vi "Rinse.vi"(8 "High pressure purge time (s)":dbl=30.0 format="%#.4f", 9 "High pressure purge?":bool=TRUE, 10 "Control parameters":T1={"Pump 2 fill rate (ml/min)"=0.5, "Pump 2 rinse times"=2, "Pump 2 fill volume (ml)"=0.015, "Pump 1 rinse rate (ml/min)"=0.2, "Pump 1 rinse volume (mL)"=1.0, "Pump 1 fill volume (mL)"=1.0, "Pump 1 fill rate (ml/min)"=3.0, "Delayed time for waiting(s)"=5.0, "Pump 3 fill rate (ml/min)"=0.5, "Pump 3 fill volume (ml)"=0.015, "Pump 3 muliplier"=1.2, "Pump 3 rinse times"=1, "Gas purge muliplier"=2.0, "Gas purge?"=TRUE, "Pump 1 clear rate (ml/min)"=0.1, "Clear?"=TRUE, "Rinse injection order"=enum."Pump 2 first"} {"Pump 1 clear rate (ml/min)" format="%#.4f"; "Gas purge muliplier" min=0.0 max=50.0 format="%#.3g"; "Pump 3 muliplier" min=0.0 max=50.0 format="%#.3g"; "Pump 3 fill volume (ml)" min=0.0 max=50.0 format="%#.3g"; "Pump 3 fill rate (ml/min)" min=0.0 max=500.0 format="%#.3g"; "Pump 1 fill rate (ml/min)" format="%#.4f"; "Pump 1 fill volume (mL)" format="%#.4f"; "Pump 1 rinse volume (mL)" format="%#.4f"; "Pump 1 rinse rate (ml/min)" format="%#.4f"; "Pump 2 fill volume (ml)" min=0.0 max=50.0 format="%#.3g"; "Pump 2 fill rate (ml/min)" min=0.0 max=500.0 format="%#.3g"}, 11 "Configured COM ports":T2={"Pump 1 COM"="COM12", "Pump 2 COM"="COM9", "Pump 3 COM"="COM13", "Pump 4 COM"="COM4", "Pump 5 COM"="COM15"}) -> ()   [LabVIEW 2017]
uses:
  <instrlib>/Harvard Apparatus PHD Ultra Series/Harvard Apparatus PHD Ultra Series.lvlib
  <instrlib>/Harvard Syringe Pump PHD2000/Harvard Syringe Pump PHD2000.lvlib
panel:
  out "Rinse injection order":enum16{"Pump 2 first", "Pump 3 first"}(ring)
  out "Clear?":bool
  out "Pump 1 clear rate (ml/min)":dbl=0.6 format="%#.4f"
  out "Gas purge?":bool
  out "Gas purge muliplier":dbl=1.2 min=0.0 max=50.0 format="%#.3g"
  out "Pump 3 rinse times":i32=2
  out "Pump 3 muliplier":dbl=1.2 min=0.0 max=50.0 format="%#.3g"
  out "Rinse injection selector":enum16{"Pump 2", "Pump 3"}(ring)
  out "Pump 3 fill volume (ml)":dbl=0.1 min=0.0 max=50.0 format="%#.3g"
  out "Pump 3 fill rate (ml/min)":dbl=0.5 min=0.0 max=500.0 format="%#.3g"
  out "Pump 5 COM":refnum<visa-resource-name>="COM12"
  out "Pump 1 rinse volume (mL)":dbl=0.4 format="%#.4f"
  out "Pump 1 rinse rate (ml/min)":dbl=0.6 format="%#.4f"
  out "Delayed time for waiting(s)":dbl
  out "Pump 1 fill volume (mL)":dbl=0.4 format="%#.4f"
  out "Pump 1 fill rate (ml/min)":dbl=1.5 format="%#.4f"
  out "Counter":i32
  out "Action selector":enum16{"Fill", "Rinse", "Clear"}(ring)
  out "Pump 2 rinse times":i32=2
  out "Pump 2 fill volume (ml)":dbl=0.1 min=0.0 max=50.0 format="%#.3g"
  out "Pump 2 fill rate (ml/min)":dbl=0.5 min=0.0 max=500.0 format="%#.3g"
  out "Pump 4 COM":refnum<visa-resource-name>="COM12"
  out "Pump 3 COM":refnum<visa-resource-name>="COM12"
  out "Pump 2 COM":refnum<visa-resource-name>="COM12"
  out "Pump 1 COM":refnum<visa-resource-name>="COM12"
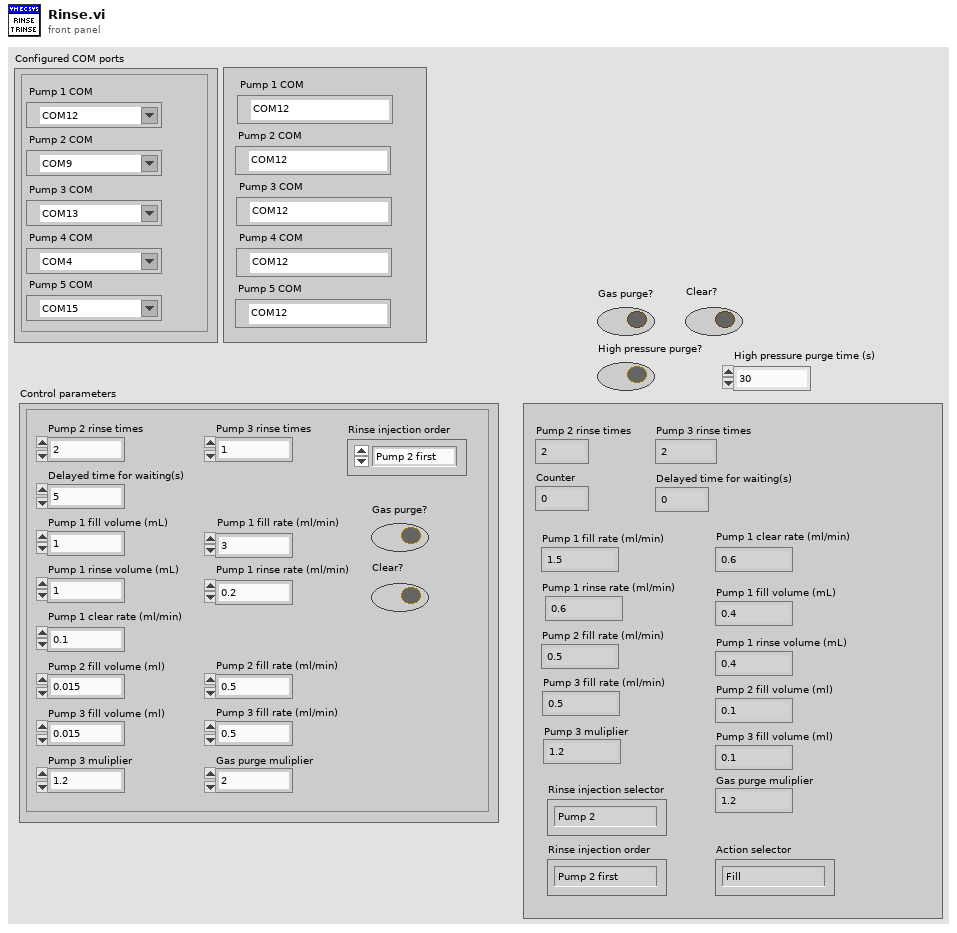
[diagram p1: front panel]
types:
  T1 = cluster{"Pump 2 fill rate (ml/min)":dbl, "Pump 2 rinse times":i32, "Pump 2 fill volume (ml)":dbl, "Pump 1 rinse rate (ml/min)":dbl, "Pump 1 rinse volume (mL)":dbl, "Pump 1 fill volume (mL)":dbl, "Pump 1 fill rate (ml/min)":dbl, "Delayed time for waiting(s)":dbl, "Pump 3 fill rate (ml/min)":dbl, "Pump 3 fill volume (ml)":dbl, "Pump 3 muliplier":dbl, "Pump 3 rinse times":i32, "Gas purge muliplier":dbl, "Gas purge?":bool, "Pump 1 clear rate (ml/min)":dbl, "Clear?":bool, "Rinse injection order":enum16{"Pump 2 first", "Pump 3 first"}}
  T2 = cluster{"Pump 1 COM":refnum<visa-resource-name>, "Pump 2 COM":refnum<visa-resource-name>, "Pump 3 COM":refnum<visa-resource-name>, "Pump 4 COM":refnum<visa-resource-name>, "Pump 5 COM":refnum<visa-resource-name>}
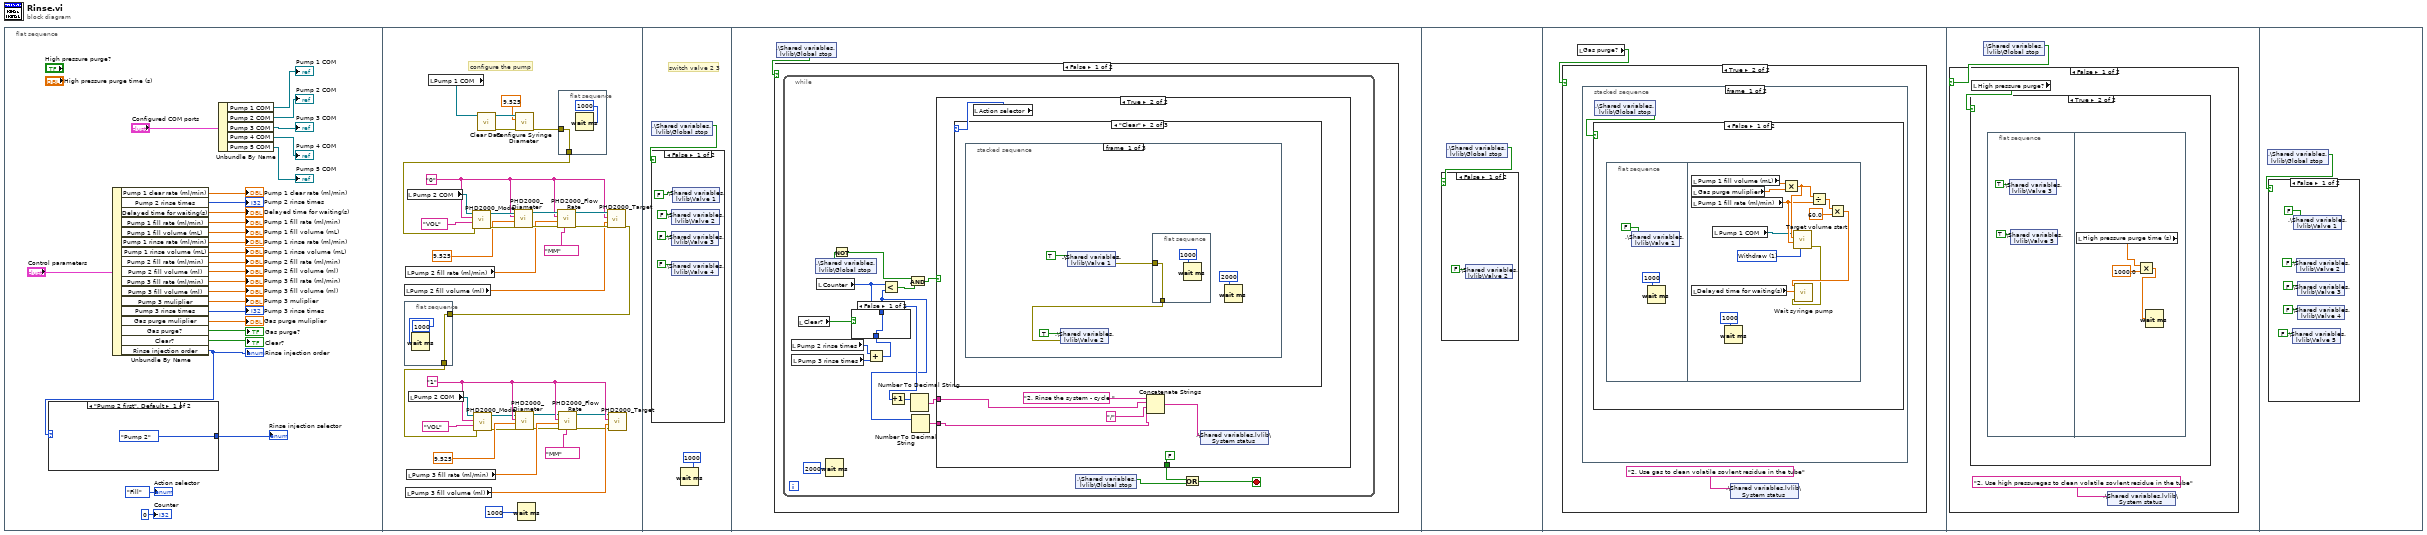
[diagram p0: block diagram]
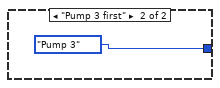
[diagram p2: hidden frame]
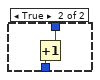
[diagram p4: hidden frame]
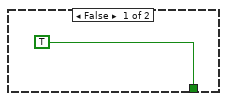
[diagram p5: hidden frame]
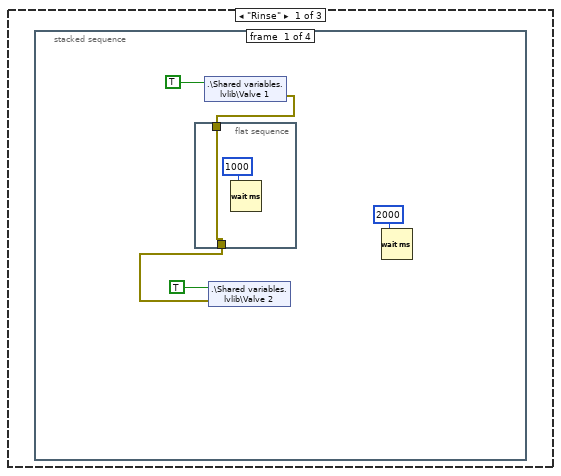
[diagram p6: hidden frame]
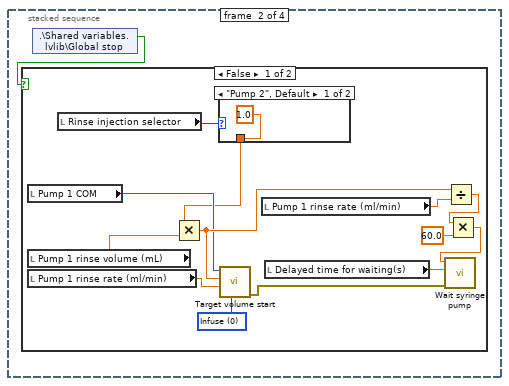
[diagram p7: hidden frame]
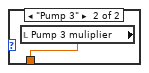
[diagram p8: hidden frame]
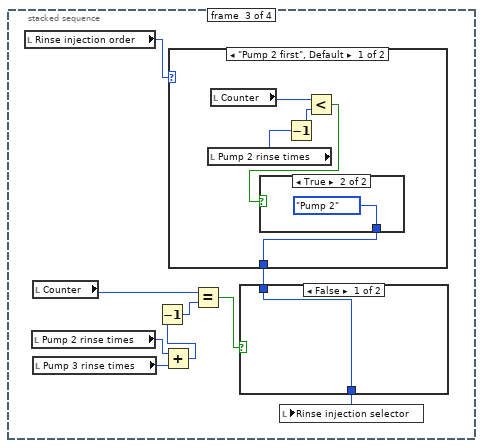
[diagram p10: hidden frame]
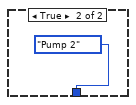
[diagram p11: hidden frame]
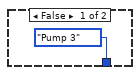
[diagram p12: hidden frame]
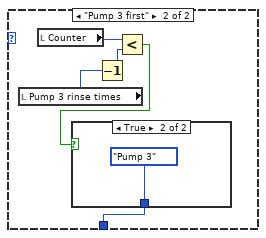
[diagram p13: hidden frame]
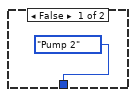
[diagram p14: hidden frame]
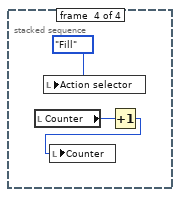
[diagram p15: hidden frame]
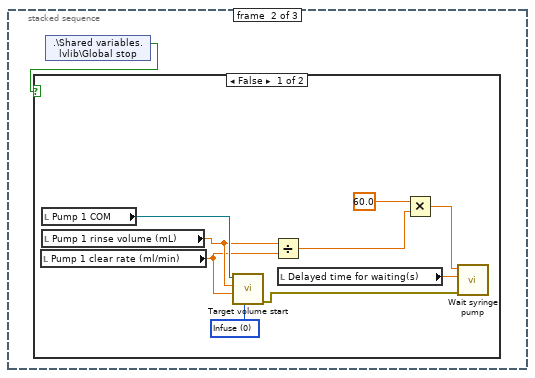
[diagram p16: hidden frame]
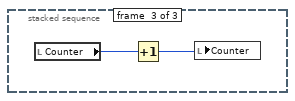
[diagram p18: hidden frame]
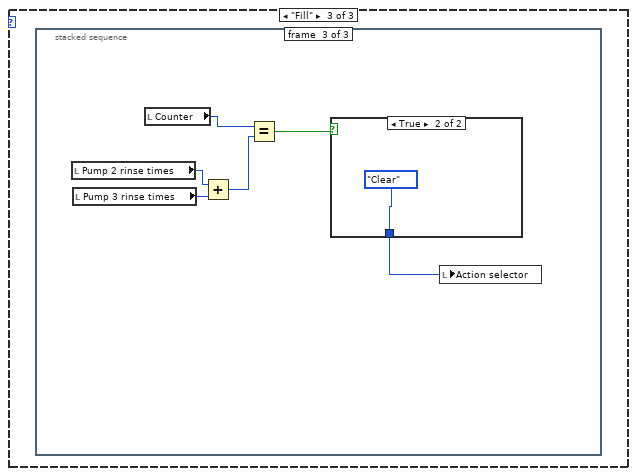
[diagram p19: hidden frame]
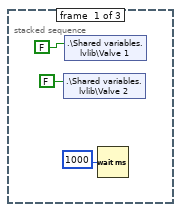
[diagram p20: hidden frame]
diagram:
  n1 = flat-sequence {
    frame #0 {
      n2 = Unbundle By Name("Control parameters") -> ("Pump 1 clear rate (ml/min)"=→"Pump 1 clear rate (ml/min)":dbl, "Pump 2 rinse times"=→"Pump 2 rinse times":i32, "Delayed time for waiting(s)"=→"Delayed time for waiting(s)":dbl, "Pump 1 fill rate (ml/min)"=→"Pump 1 fill rate (ml/min)":dbl, "Pump 1 fill volume (mL)"=→"Pump 1 fill volume (mL)":dbl, "Pump 1 rinse rate (ml/min)"=→"Pump 1 rinse rate (ml/min)":dbl, "Pump 1 rinse volume (mL)"=→"Pump 1 rinse volume (mL)":dbl, "Pump 2 fill rate (ml/min)"=→"Pump 2 fill rate (ml/min)":dbl, "Pump 2 fill volume (ml)"=→"Pump 2 fill volume (ml)":dbl, "Pump 3 fill rate (ml/min)"=→"Pump 3 fill rate (ml/min)":dbl, "Pump 3 fill volume (ml)"=→"Pump 3 fill volume (ml)":dbl, "Pump 3 muliplier"=→"Pump 3 muliplier":dbl, "Pump 3 rinse times"=→"Pump 3 rinse times":i32, "Gas purge muliplier"=→"Gas purge muliplier":dbl, "Gas purge?"=→"Gas purge?":bool, "Clear?"=→"Clear?":bool, "Rinse injection order"=w1:enum16{"Pump 2 first", "Pump 3 first"})
      "Rinse injection order" <- w1
      n3 = case shown="\"Pump 2 first\", Default" w1 {
        tunnel: [enum16{"Pump 2", "Pump 3"}."Pump 2" ("Rinse injection selector") enum16{"Pump 2", "Pump 3"}."Pump 3" ("Rinse injection selector")] -> w2
        frame "Pump 2 first", Default {
        }
        frame "Pump 3 first" {
        }
      }
      "Rinse injection selector" <- w2
      n4 = Unbundle By Name("Configured COM ports") -> ("Pump 1 COM"=→"Pump 1 COM":refnum<visa-resource-name>, "Pump 2 COM"=→"Pump 2 COM":refnum<visa-resource-name>, "Pump 3 COM"=→"Pump 3 COM":refnum<visa-resource-name>, "Pump 4 COM"=→"Pump 4 COM":refnum<visa-resource-name>, "Pump 5 COM"=→"Pump 5 COM":refnum<visa-resource-name>)
      "Action selector" <- enum16{"Fill", "Rinse", "Clear"}."Fill" ("Action selector")
      "Counter" <- 0 ("Counter")
    }
    frame #1 {
      w41 = "1" ("Pump #")
      w50 = "0" ("Pump #")
      # "configure the pump"
      n5 = local read "Pump 2 fill volume (ml)"() -> (w48:dbl)
      n6 = flat-sequence {
        tunnel: w44 -> [w65]
        tunnel: [w65] -> w30
        frame #0 {
          n7 = Wait (ms)(milliseconds to wait=u32 1000) -> ()  [unwired: 1 out]
        }
      }
      n8 = local read "Pump 2 fill rate (ml/min)"() -> (w49:dbl)
      n9 = local read "Pump 3 fill volume (ml)"() -> (w43:dbl)
      n10 = local read "Pump 3 fill rate (ml/min)"() -> (w42:dbl)
      n11 = local read "Pump 2 COM"() -> (w55:refnum<visa-resource-name>)
      n12 = local read "Pump 2 COM"() -> (w36:refnum<visa-resource-name>)
      n13 = local read "Pump 1 COM"() -> (w57:refnum<visa-resource-name>)
      n14 = call <instrlib>:"PHD2000_Mode.vi"("error in (no error)"=w46, "Mode"="VOL", "Pump #"=w50, "VISA resource name 2"=w55) -> ("error out"=w53:errorcluster, "VISA resource name out"=w54:refnum<visa-resource-name>)  [unwired: 5 in, 1 out]
      n15 = call <instrlib>:"PHD2000_Mode.vi"("error in (no error)"=w30, "Mode"="VOL", "Pump #"=w41, "VISA resource name 2"=w36) -> ("error out"=w38:errorcluster, "VISA resource name out"=w37:refnum<visa-resource-name>)  [unwired: 5 in, 1 out]
      n16 = call <instrlib>:"Clear Data.vi"("VISA resource name"=w57) -> ("error out"=w59:errorcluster, "VISA resource name out"=w58:refnum<visa-resource-name>)  [unwired: 9 in]
      n17 = call <instrlib>:"PHD2000_Diameter.vi"("VISA resource name 2"=w54, "Pump #"=w50, "diameter (mm)"=9.525 ("Syringe Diameter (20 mm)"), "error in (no error)"=w53) -> ("VISA resource name out"=w61:refnum<visa-resource-name>, "error out"=w63:errorcluster)  [unwired: 5 in]
      n18 = call <instrlib>:"Configure Syringe Diameter.vi"("error in (no error)"=w59, "Syringe Diameter (20 mm)"=9.525, "VISA resource name"=w58) -> ("error out"=w45:errorcluster)  [unwired: 7 in, 1 out]
      n19 = call <instrlib>:"PHD2000_Diameter.vi"("VISA resource name 2"=w37, "Pump #"=w41, "diameter (mm)"=9.525 ("Syringe Diameter (20 mm)"), "error in (no error)"=w38) -> ("VISA resource name out"=w34:refnum<visa-resource-name>, "error out"=w32:errorcluster)  [unwired: 5 in]
      n20 = Wait (ms)(milliseconds to wait=u32 1000) -> ()  [unwired: 1 out]
      n21 = call <instrlib>:"PHD2000_Flow Rate.vi"("VISA resource name 2"=w61, "Pump #"=w50, "flowrate"=w49, "error in (no error)"=w63, "Unit"="MM") -> ("VISA resource name out"=w62:refnum<visa-resource-name>, "error out"=w64:errorcluster)  [unwired: 4 in]
      n22 = flat-sequence {
        tunnel: [w67] -> w46
        tunnel: w45 -> [w67]
        frame #0 {
          n23 = Wait (ms)(milliseconds to wait=u32 1000) -> ()  [unwired: 1 out]
        }
      }
      n24 = call <instrlib>:"PHD2000_Flow Rate.vi"("VISA resource name 2"=w34, "Pump #"=w41, "flowrate"=w42, "error in (no error)"=w32, "Unit"="MM") -> ("VISA resource name out"=w33:refnum<visa-resource-name>, "error out"=w31:errorcluster)  [unwired: 4 in]
      n25 = call <instrlib>:"PHD2000_Target.vi"("error in (no error)"=w64, "Target (ml)"=w48, "Pump #"=w50, "VISA resource name 2"=w62) -> ("error out"=w44:errorcluster)  [unwired: 5 in, 2 out]
      n26 = call <instrlib>:"PHD2000_Target.vi"("error in (no error)"=w31, "Target (ml)"=w43, "Pump #"=w41, "VISA resource name 2"=w33) -> ()  [unwired: 5 in, 3 out]
    }
    frame #2 {
      # "switch valve 2 3"
      n27 = shared-variable ".\\Shared variables.lvlib\\Global stop"() -> (w70:bool)  [unwired: 1 in, 1 out]
      n28 = case shown="False" w70 {
        frame False {
          n29 = shared-variable ".\\Shared variables.lvlib\\Valve 3"(FALSE ("Valve 3")) -> ()  [unwired: 1 in, 1 out]
          n30 = shared-variable ".\\Shared variables.lvlib\\Valve 4"(FALSE ("Valve 3")) -> ()  [unwired: 1 in, 1 out]
          n31 = shared-variable ".\\Shared variables.lvlib\\Valve 2"(FALSE ("Valve 2")) -> ()  [unwired: 1 in, 1 out]
          n32 = shared-variable ".\\Shared variables.lvlib\\Valve 1"(FALSE ("Valve 1")) -> ()  [unwired: 1 in, 1 out]
        }
        frame True {
        }
      }
      n33 = Wait (ms)(milliseconds to wait=u32 1000) -> ()  [unwired: 1 out]
    }
    frame #3 {
      n34 = shared-variable ".\\Shared variables.lvlib\\Global stop"() -> (w75:bool)  [unwired: 1 in, 1 out]
      n35 = case shown="False" w75 {
        frame False {
          n36 = while {
            stop <- w91 stop-if-true
            n37 = local read "Pump 2 rinse times"() -> (w82:i32)
            n38 = local read "Pump 3 rinse times"() -> (w81:i32)
            n39 = local read "Clear?"() -> (w84:bool)
            n40 = shared-variable ".\\Shared variables.lvlib\\Global stop"() -> (w88:bool)  [unwired: 1 in, 1 out]
            n41 = local read "Counter"() -> (w79:i32)
            n42 = Wait (ms)(milliseconds to wait=u32 2000) -> ()  [unwired: 1 out]
            n43 = Not(x=w88) -> (.not. x?=w85:bool)
            n44 = Add(x=w82, y=w81) -> (x+y=w83:i32)
            n45 = case shown="False" w84 {
              tunnel: w83 -> [w93 w95]
              tunnel: [w93 w94] -> w78
              frame False {
              }
              frame True {
                n46 = Increment(x=w95) -> (x+1=w94:i32)
              }
            }
            n47 = Less?(x=w79, y=w78) -> (x < y?=w86:bool)
            n48 = Increment(x=w79) -> (x+1=w80:i32)
            n49 = And(x=w85, y=w86) -> (x .and. y?=w87:bool)
            n50 = Number To Decimal String(number=w80) -> (decimal integer string=w77:string)  [unwired: 1 in]
            n51 = Number To Decimal String(number=w78) -> (decimal integer string=w76:string)  [unwired: 1 in]
            n52 = case shown="True" w87 {
              tunnel: [TRUE FALSE] -> w90
              tunnel: w77 -> [_ w98]
              tunnel: w76 -> [_ w97]
              frame False {
              }
              frame True {
                n53 = local read "Action selector"() -> (w103:enum16{"Fill", "Rinse", "Clear"})
                n54 = case shown="\"Clear\"" w103 {
                  frame "Rinse" {
                    n55 = stacked-sequence {
                      frame #0 {
                        n56 = flat-sequence {
                          tunnel: w105 -> [w109]
                          tunnel: [w109] -> w104
                          frame #0 {
                            n57 = Wait (ms)(milliseconds to wait=u32 1000) -> ()  [unwired: 1 out]
                          }
                        }
                        n58 = shared-variable ".\\Shared variables.lvlib\\Valve 1"(TRUE ("Valve 1")) -> (error out=w105:errorcluster)  [unwired: 1 in]
                        n59 = shared-variable ".\\Shared variables.lvlib\\Valve 2"(TRUE ("Valve 1"), error in=w104) -> ()  [unwired: 1 out]
                        n60 = Wait (ms)(milliseconds to wait=u32 2000) -> ()  [unwired: 1 out]
                      }
                      frame #1 {
                        n61 = shared-variable ".\\Shared variables.lvlib\\Global stop"() -> (w111:bool)  [unwired: 1 in, 1 out]
                        n62 = case shown="False" w111 {
                          frame False {
                            w119 = u16 0 items=["Infuse", "Withdraw"] ("Pump Direction (0:Infuse)")
                            n63 = local read "Pump 1 COM"() -> (w120:refnum<visa-resource-name>)
                            n64 = local read "Pump 1 rinse volume (mL)"() -> (w117:dbl)
                            n65 = local read "Pump 1 rinse rate (ml/min)"() -> (w118:dbl)
                            n66 = local read "Rinse injection selector"() -> (w112:enum16{"Pump 2", "Pump 3"})
                            n67 = case shown="\"Pump 2\", Default" w112 {
                              tunnel: [1.0 ("y") w126] -> w116
                              frame "Pump 2", Default {
                              }
                              frame "Pump 3" {
                                n68 = local read "Pump 3 muliplier"() -> (w126:dbl)
                              }
                            }
                            n69 = Multiply(x=w116, y=w117) -> (x*y=w121:dbl)
                            n70 = call "Target volume start.vi"("Pump Direction (0:Infuse)"=w119, "Flow Rate (ml/min)"=w118, "Target volume (ml)"=w121, "VISA resource name"=w120) -> ("error out"=w113:errorcluster)  [unwired: 6 in, 1 out]
                            n71 = local read "Pump 1 rinse rate (ml/min)"() -> (w124:dbl)
                            n72 = local read "Delayed time for waiting(s)"() -> (w114:dbl)
                            n73 = Divide(x=w121, y=w124) -> (x/y=w123:dbl)
                            n74 = Multiply(x=w123, y=60.0) -> (x*y=w115:dbl)
                            n75 = call "Wait syringe pump.vi"("error in (no error)"=w113, "Delayed time (s)"=w114, "Time Target (s)"=w115) -> ()  [unwired: 8 in, 1 out]
                          }
                          frame True {
                          }
                        }
                      }
                      frame #2 {
                        n76 = local read "Rinse injection order"() -> (w135:enum16{"Pump 2 first", "Pump 3 first"})
                        n77 = local read "Pump 2 rinse times"() -> (w134:i32)
                        n78 = local read "Counter"() -> (w130:i32)
                        n79 = local read "Pump 3 rinse times"() -> (w133:i32)
                        n80 = Add(x=w134, y=w133) -> (x+y=w132:i32)
                        n81 = Decrement(x=w132) -> (x-1=w131:i32)
                        n82 = case shown="\"Pump 2 first\", Default" w135 {
                          tunnel: [w138 w145] -> w127
                          frame "Pump 2 first", Default {
                            n83 = local read "Pump 2 rinse times"() -> (w141:i32)
                            n84 = local read "Counter"() -> (w142:i32)
                            n85 = Decrement(x=w141) -> (x-1=w140:i32)
                            n86 = Less?(x=w142, y=w140) -> (x < y?=w139:bool)
                            n87 = case shown="True" w139 {
                              tunnel: [enum16{"Pump 2", "Pump 3"}."Pump 3" ("Rinse injection selector") enum16{"Pump 2", "Pump 3"}."Pump 2" ("Rinse injection selector")] -> w138
                              frame False {
                              }
                              frame True {
                              }
                            }
                          }
                          frame "Pump 3 first" {
                            n88 = local read "Pump 3 rinse times"() -> (w148:i32)
                            n89 = local read "Counter"() -> (w149:i32)
                            n90 = Decrement(x=w148) -> (x-1=w147:i32)
                            n91 = Less?(x=w149, y=w147) -> (x < y?=w146:bool)
                            n92 = case shown="True" w146 {
                              tunnel: [enum16{"Pump 2", "Pump 3"}."Pump 2" ("Rinse injection selector") enum16{"Pump 2", "Pump 3"}."Pump 3" ("Rinse injection selector")] -> w145
                              frame False {
                              }
                              frame True {
                              }
                            }
                          }
                        }
                        n93 = Equal?(x=w130, y=w131) -> (x = y?=w129:bool)
                        n94 = case shown="False" w129 {
                          tunnel: [w136 enum16{"Pump 2", "Pump 3"}."Pump 2" ("Rinse injection selector")] -> w128
                          tunnel: w127 -> [w136 _]
                          frame False {
                          }
                          frame True {
                          }
                        }
                        n95 = local write "Rinse injection selector"(w128) -> ()
                      }
                      frame #3 {
                        n96 = local read "Counter"() -> (w154:i32)
                        n97 = local write "Action selector"(enum16{"Fill", "Rinse", "Clear"}."Fill" ("Action selector")) -> ()
                        n98 = Increment(x=w154) -> (x+1=w153:i32)
                        n99 = local write "Counter"(w153) -> ()
                      }
                    }
                  }
                  frame "Clear" {
                    n100 = stacked-sequence {
                      frame #0 {
                        n101 = shared-variable ".\\Shared variables.lvlib\\Valve 2"(TRUE ("Valve 1"), error in=w157) -> ()  [unwired: 1 out]
                        n102 = shared-variable ".\\Shared variables.lvlib\\Valve 1"(TRUE ("Valve 1")) -> ()  [unwired: 1 in, 1 out]
                        n103 = shared-variable ".\\Shared variables.lvlib\\Valve 1"(TRUE ("Valve 1")) -> (error out=w156:errorcluster)  [unwired: 1 in]
                        n104 = flat-sequence {
                          tunnel: [w161] -> w157
                          tunnel: w156 -> [w161]
                          frame #0 {
                            n105 = Wait (ms)(milliseconds to wait=u32 1000) -> ()  [unwired: 1 out]
                          }
                        }
                        n106 = Wait (ms)(milliseconds to wait=u32 2000) -> ()  [unwired: 1 out]
                      }
                      frame #1 {
                        n107 = shared-variable ".\\Shared variables.lvlib\\Global stop"() -> (w163:bool)  [unwired: 1 in, 1 out]
                        n108 = case shown="False" w163 {
                          frame False {
                            w171 = u16 0 items=["Infuse", "Withdraw"] ("Pump Direction (0:Infuse)")
                            n109 = local read "Pump 1 clear rate (ml/min)"() -> (w166:dbl)
                            n110 = local read "Pump 1 COM"() -> (w172:refnum<visa-resource-name>)
                            n111 = local read "Pump 1 rinse volume (mL)"() -> (w167:dbl)
                            n112 = call "Target volume start.vi"("Pump Direction (0:Infuse)"=w171, "Flow Rate (ml/min)"=w166, "Target volume (ml)"=w167, "VISA resource name"=w172) -> ("error out"=w168:errorcluster)  [unwired: 6 in, 1 out]
                            n113 = Divide(x=w167, y=w166) -> (x/y=w164:dbl)
                            n114 = local read "Delayed time for waiting(s)"() -> (w169:dbl)
                            n115 = Multiply(x=60.0 ("y"), y=w164) -> (x*y=w170:dbl)
                            n116 = call "Wait syringe pump.vi"("error in (no error)"=w168, "Delayed time (s)"=w169, "Time Target (s)"=w170) -> ()  [unwired: 8 in, 1 out]
                          }
                          frame True {
                          }
                        }
                      }
                      frame #2 {
                        n117 = local read "Counter"() -> (w174:i32)
                        n118 = Increment(x=w174) -> (x+1=w173:i32)
                        n119 = local write "Counter"(w173) -> ()
                      }
                    }
                  }
                  frame "Fill" {
                    n120 = stacked-sequence {
                      frame #0 {
                        n121 = shared-variable ".\\Shared variables.lvlib\\Valve 2"(FALSE ("Valve 2")) -> ()  [unwired: 1 in, 1 out]
                        n122 = shared-variable ".\\Shared variables.lvlib\\Valve 1"(FALSE ("Valve 1")) -> ()  [unwired: 1 in, 1 out]
                        n123 = Wait (ms)(milliseconds to wait=u32 1000) -> ()  [unwired: 1 out]
                      }
                      frame #1 {
                        n124 = shared-variable ".\\Shared variables.lvlib\\Global stop"() -> (w178:bool)  [unwired: 1 in, 1 out]
                        n125 = case shown="False" w178 {
                          frame False {
                            w185 = u16 1 items=["Infuse", "Withdraw"] ("Pump Direction (0:Infuse)")
                            n126 = local read "Rinse injection selector"() -> (w191:enum16{"Pump 2", "Pump 3"})
                            n127 = case shown="\"Pump 3\"" w191 {
                              tunnel: [w196 w203] -> w179
                              tunnel: [1.0 ("Pump 3 muliplier") w207] -> w184
                              tunnel: [w197 w204] -> w182
                              frame "Pump 2", Default {
                                n128 = local read "Pump 2 fill volume (ml)"() -> (w199:dbl)
                                n129 = local read "Pump 2 fill rate (ml/min)"() -> (w198:dbl)
                                n130 = local read "Pump 2 COM"() -> (w195:refnum<visa-resource-name>)
                                n131 = call "PHD2000 RUN SURE.vi"("Pump #"="0", "VISA resource name 2"=w195) -> ("error out"=w196:errorcluster)  [unwired: 8 in, 1 out]
                                n132 = Divide(x=w199, y=w198) -> (x/y=w197:dbl)
                              }
                              frame "Pump 3" {
                                n133 = local read "Pump 3 fill rate (ml/min)"() -> (w205:dbl)
                                n134 = local read "Pump 3 muliplier"() -> (w207:dbl)
                                n135 = local read "Pump 3 fill volume (ml)"() -> (w206:dbl)
                                n136 = local read "Pump 2 COM"() -> (w201:refnum<visa-resource-name>)
                                n137 = Divide(x=w206, y=w205) -> (x/y=w204:dbl)
                                n138 = call "PHD2000 RUN SURE.vi"("Pump #"="1", "VISA resource name 2"=w201) -> ("error out"=w203:errorcluster)  [unwired: 8 in, 1 out]
                              }
                            }
                            n139 = local read "Pump 1 fill volume (mL)"() -> (w186:dbl)
                            n140 = local read "Pump 1 COM"() -> (w187:refnum<visa-resource-name>)
                            n141 = local read "Pump 1 fill rate (ml/min)"() -> (w188:dbl)
                            n142 = local read "Pump 1 fill rate (ml/min)"() -> (w190:dbl)
                            n143 = Multiply(x=w184, y=w186) -> (x*y=w189:dbl)
                            n144 = call "Target volume start.vi"("Pump Direction (0:Infuse)"=w185, "Flow Rate (ml/min)"=w188, "Target volume (ml)"=w189, "VISA resource name"=w187) -> ()  [unwired: 6 in, 2 out]
                            n145 = Divide(x=w189, y=w190) -> (x/y=w183:dbl)
                            n146 = local read "Delayed time for waiting(s)"() -> (w192:dbl)
                            n147 = Max & Min(x=w182, y=w183) -> (max(x,y)=w181:dbl)  [unwired: 1 out]
                            n148 = Multiply(x=w181, y=60.0) -> (x*y=w193:dbl)
                            n149 = call "Wait syringe pump.vi"("error in (no error)"=w179, "Delayed time (s)"=w192, "Time Target (s)"=w193) -> ()  [unwired: 8 in, 1 out]
                          }
                          frame True {
                          }
                        }
                      }
                      frame #2 {
                        n150 = local read "Pump 2 rinse times"() -> (w209:i32)
                        n151 = local read "Pump 3 rinse times"() -> (w208:i32)
                        n152 = local read "Counter"() -> (w213:i32)
                        n153 = Add(x=w209, y=w208) -> (x+y=w212:i32)
                        n154 = Equal?(x=w213, y=w212) -> (x = y?=w211:bool)
                        n155 = case shown="True" w211 {
                          tunnel: [enum16{"Fill", "Rinse", "Clear"}."Rinse" ("Action selector") enum16{"Fill", "Rinse", "Clear"}."Clear" ("Action selector")] -> w210
                          frame False {
                          }
                          frame True {
                          }
                        }
                        n156 = local write "Action selector"(w210) -> ()
                      }
                    }
                  }
                }
                n157 = Concatenate Strings("2. Rinse the system - cycle " ("System status"), w98, "/" ("string"), w97) -> (w101:string)
                n158 = shared-variable ".\\Shared variables.lvlib\\System status"(w101) -> ()  [unwired: 1 in, 1 out]
              }
            }
            n159 = shared-variable ".\\Shared variables.lvlib\\Global stop"() -> (w92:bool)  [unwired: 1 in, 1 out]
            n160 = Or(x=w90, y=w92) -> (x .or. y?=w91:bool)
          }
        }
        frame True {
        }
      }
    }
    frame #4 {
      n161 = shared-variable ".\\Shared variables.lvlib\\Global stop"() -> (w216:bool)  [unwired: 1 in, 1 out]
      n162 = case shown="False" w216 {
        frame False {
          n163 = shared-variable ".\\Shared variables.lvlib\\Valve 2"(FALSE ("Valve 2")) -> ()  [unwired: 1 in, 1 out]
        }
        frame True {
        }
      }
    }
    frame #5 {
      n164 = local read "Gas purge?"() -> (w218:bool)
      n165 = case shown="True" w218 {
        frame False {
        }
        frame True {
          n166 = stacked-sequence {
            frame #0 {
              n167 = shared-variable ".\\Shared variables.lvlib\\Global stop"() -> (w220:bool)  [unwired: 1 in, 1 out]
              n168 = case shown="False" w220 {
                frame False {
                  n169 = flat-sequence {
                    frame #0 {
                      n170 = shared-variable ".\\Shared variables.lvlib\\Valve 1"(FALSE ("Valve 1")) -> ()  [unwired: 1 in, 1 out]
                      n171 = Wait (ms)(milliseconds to wait=u32 1000) -> ()  [unwired: 1 out]
                    }
                    frame #1 {
                      w227 = u16 1 items=["Infuse", "Withdraw"] ("Pump Direction (0:Infuse)")
                      n172 = local read "Delayed time for waiting(s)"() -> (w225:dbl)
                      n173 = local read "Pump 1 fill volume (mL)"() -> (w229:dbl)
                      n174 = local read "Gas purge muliplier"() -> (w226:dbl)
                      n175 = local read "Pump 1 fill rate (ml/min)"() -> (w233:dbl)
                      n176 = local read "Pump 1 COM"() -> (w230:refnum<visa-resource-name>)
                      n177 = Wait (ms)(milliseconds to wait=u32 1000) -> ()  [unwired: 1 out]
                      n178 = Multiply(x=w229, y=w226) -> (x*y=w234:dbl)
                      n179 = call "Target volume start.vi"("Pump Direction (0:Infuse)"=w227, "Flow Rate (ml/min)"=w233, "Target volume (ml)"=w234, "VISA resource name"=w230) -> ("error out"=w223:errorcluster)  [unwired: 6 in, 1 out]
                      n180 = Divide(x=w234, y=w233) -> (x/y=w231:dbl)
                      n181 = Multiply(x=w231, y=60.0) -> (x*y=w224:dbl)
                      n182 = call "Wait syringe pump.vi"("error in (no error)"=w223, "Delayed time (s)"=w225, "Time Target (s)"=w224) -> ()  [unwired: 8 in, 1 out]
                    }
                  }
                }
                frame True {
                }
              }
            }
            frame #1 {
              n183 = shared-variable ".\\Shared variables.lvlib\\Global stop"() -> (w235:bool)  [unwired: 1 in, 1 out]
              n184 = case shown="False" w235 {
                frame False {
                  n185 = flat-sequence {
                    frame #0 {
                      n186 = shared-variable ".\\Shared variables.lvlib\\Valve 1"(TRUE ("Valve 1")) -> ()  [unwired: 1 in, 1 out]
                      n187 = Wait (ms)(milliseconds to wait=u32 1000) -> ()  [unwired: 1 out]
                    }
                    frame #1 {
                      w245 = u16 0 items=["Infuse", "Withdraw"] ("Pump Direction (0:Infuse)")
                      n188 = local read "Pump 1 rinse volume (mL)"() -> (w247:dbl)
                      n189 = local read "Pump 1 rinse rate (ml/min)"() -> (w239:dbl)
                      n190 = local read "Gas purge muliplier"() -> (w240:dbl)
                      n191 = local read "Delayed time for waiting(s)"() -> (w244:dbl)
                      n192 = local read "Pump 1 COM"() -> (w248:refnum<visa-resource-name>)
                      n193 = Wait (ms)(milliseconds to wait=u32 1000) -> ()  [unwired: 1 out]
                      n194 = Multiply(x=w247, y=w240) -> (x*y=w241:dbl)
                      n195 = Multiply(x=w240, y=w239) -> (x*y=w238:dbl)
                      n196 = call "Target volume start.vi"("Pump Direction (0:Infuse)"=w245, "Flow Rate (ml/min)"=w238, "Target volume (ml)"=w241, "VISA resource name"=w248) -> ("error out"=w242:errorcluster)  [unwired: 6 in, 1 out]
                      n197 = Divide(x=w241, y=w238) -> (x/y=w249:dbl)
                      n198 = Multiply(x=w249, y=60.0) -> (x*y=w243:dbl)
                      n199 = call "Wait syringe pump.vi"("error in (no error)"=w242, "Delayed time (s)"=w244, "Time Target (s)"=w243) -> ()  [unwired: 8 in, 1 out]
                    }
                  }
                }
                frame True {
                }
              }
            }
          }
          n200 = shared-variable ".\\Shared variables.lvlib\\System status"("2. Use gas to clean volatile sovlent residue in the tube" ("System status")) -> ()  [unwired: 1 in, 1 out]
        }
      }
    }
    frame #6 {
      n201 = shared-variable ".\\Shared variables.lvlib\\Global stop"() -> (w251:bool)  [unwired: 1 in, 1 out]
      n202 = case shown="False" w251 {
        frame False {
          n203 = local read "High pressure purge?"() -> (w252:bool)
          n204 = case shown="True" w252 {
            frame False {
            }
            frame True {
              n205 = flat-sequence {
                frame #0 {
                  n206 = shared-variable ".\\Shared variables.lvlib\\Valve 3"(TRUE ("Valve 3")) -> ()  [unwired: 1 in, 1 out]
                  n207 = shared-variable ".\\Shared variables.lvlib\\Valve 5"(TRUE ("Valve 5")) -> ()  [unwired: 1 in, 1 out]
                }
                frame #1 {
                  n208 = local read "High pressure purge time (s)"() -> (w257:dbl)
                  n209 = Multiply(x=w257, y=1000.0) -> (x*y=w256:dbl)
                  n210 = Wait (ms)(milliseconds to wait=w256) -> ()  [unwired: 1 out]
                }
              }
            }
          }
          n211 = shared-variable ".\\Shared variables.lvlib\\System status"("2. Use high pressuregas to clean volatile sovlent residue in the tube" ("System status")) -> ()  [unwired: 1 in, 1 out]
        }
        frame True {
        }
      }
    }
    frame #7 {
      n212 = shared-variable ".\\Shared variables.lvlib\\Global stop"() -> (w259:bool)  [unwired: 1 in, 1 out]
      n213 = case shown="False" w259 {
        frame False {
          n214 = shared-variable ".\\Shared variables.lvlib\\Valve 5"(FALSE ("Valve 5")) -> ()  [unwired: 1 in, 1 out]
          n215 = shared-variable ".\\Shared variables.lvlib\\Valve 1"(FALSE ("Valve 1")) -> ()  [unwired: 1 in, 1 out]
          n216 = shared-variable ".\\Shared variables.lvlib\\Valve 2"(FALSE ("Valve 2")) -> ()  [unwired: 1 in, 1 out]
          n217 = shared-variable ".\\Shared variables.lvlib\\Valve 3"(FALSE ("Valve 3")) -> ()  [unwired: 1 in, 1 out]
          n218 = shared-variable ".\\Shared variables.lvlib\\Valve 4"(FALSE ("Valve 3")) -> ()  [unwired: 1 in, 1 out]
        }
        frame True {
        }
      }
    }
  }
